vi "Teleop.vi"(0 "Call Context":T9) -> (6 "SubState 3":T4, 9 "SubState 4":T8, 11 "Loop 3 Data":T3, 14 "SubState 0":T4=enum."driver control", 15 "Loop 1 Data":T6, 16 "Loop 0 Data":T7, 17 "SubState 1":T4, 18 "Loop 2 Data":T5, 19 "SubState 2":T4)   [LabVIEW 2013]
uses:
  typedefs/subStates.ctl
  <vilib>/Rock Robotics/WPI/DriverStation/WPI_DriverStationDerivedRobotMode.ctl
  typedefs/singleUseSubstate.ctl
  typedefs/Loop Datatypes/Loop 0 Datatype.ctl
  typedefs/Loop Datatypes/Loop 1 Datatype.ctl
  typedefs/Loop Datatypes/Loop 2 Datatype.ctl
  typedefs/Loop Datatypes/Loop 3 Datatype.ctl
  <vilib>/Rock Robotics/WPI/Joystick/WPI_JoystickDevRef.ctl
  <vilib>/Rock Robotics/WPI/Joystick/WPI_JoystickDeviceEnum.ctl
  typedefs/fg_typedef.ctl
  typedefs/vision enable.ctl
  <vilib>/Rock Robotics/WPI/Joystick/WPI_JoystickGetSetRefNum.vi
panel:
  out "JS3":T1
  out "Drive to DC":bool
  out "JS1":T1
  out "JS2":T1
  out "Exit Value":i32=-1
  # "Loop Data and Substates"
  # "Drive Loop"
  # "State Machine Master Loop"
  # "Pickup/Passing Belts Loop"
  # "Pickup/Passing Arm Loop"
  # "Pneumatics Loop"
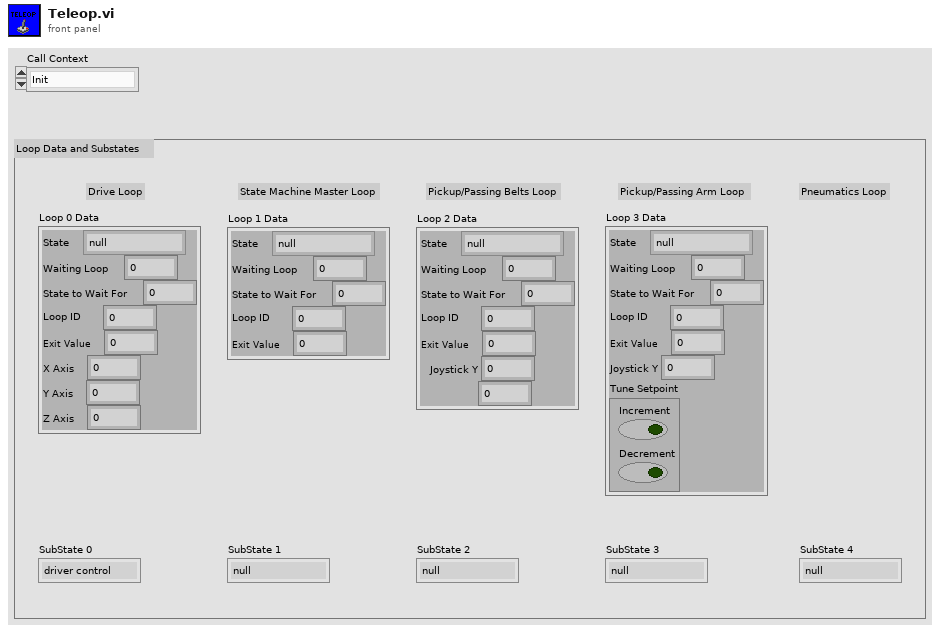
[diagram p1: front panel]
types:
  T1 = typedef "WPI_JoystickDevRef.ctl" = cluster{"Device":T2}
  T2 = typedef "WPI_JoystickDeviceEnum.ctl" = enum16{"USB 1", "USB 2", "USB 3", "USB 4", "Kinect 1", "Kinect 2"}
  T3 = typedef "Loop 3 Datatype.ctl" = cluster{"State":T4, "Waiting Loop":i32, "State to Wait For":i32, "Loop ID":i32, "Exit Value":i32, "Joystick Y":dbl, "Tune Setpoint":cluster{"Increment":bool, "Decrement":bool}}
  T4 = typedef "subStates.ctl" = enum16{"null", "wait", "driver control", "auto", "manual override", "hold position", "rotate", "pickup", "pass", "load", "goto shoot", "shoot high goal", "shoot low goal", "cancel arm", "cancel shooter", "end"}
  T5 = typedef "Loop 2 Datatype.ctl" = cluster{"State":T4, "Waiting Loop":i32, "State to Wait For":i32, "Loop ID":i32, "Exit Value":i32, "Joystick Y":dbl, "Joystick Z":dbl}
  T6 = typedef "Loop 1 Datatype.ctl" = cluster{"State":T4, "Waiting Loop":i32, "State to Wait For":i32, "Loop ID":i32, "Exit Value":i32}
  T7 = typedef "Loop 0 Datatype.ctl" = cluster{"State":T4, "Waiting Loop":i32, "State to Wait For":i32, "Loop ID":i32, "Exit Value":i32, "X Axis":dbl, "Y Axis":dbl, "Z Axis":dbl}
  T8 = typedef "singleUseSubstate.ctl" = enum16{"null", "wait", "shift high", "shift low", "extend shooter", "retract shooter", "latch", "unlatch"}
  T9 = typedef "WPI_DriverStationDerivedRobotMode.ctl" = enum16{"Init", "Execute", "Stop"}
  T10 = cluster{"axis 1 (x)":dbl, "axis 2 (y)":dbl, "axis 3 (throttle)":dbl, "axis 4":dbl, "axis 5":dbl, "axis 6":dbl}
  T11 = typedef "WPI_EncoderDevRef.ctl" = cluster{"DevStatus":errorcluster, "EncoderIndex":T12, "CounterIndex":T13, "DistancePerCount":dbl, "Decoding Type":T14}
  T12 = typedef "FPGA_EncoderIdx.ctl" = enum8{"Enc 0", "Enc 1", "Enc 2", "Enc 3", "Invalid"}
  T13 = typedef "FPGA_CounterCtrSystemIndex.ctl" = enum8{"Ctr 0", "Ctr 1", "Ctr 2", "Ctr 3", "Ctr 4", "Ctr 5", "Ctr 6", "Ctr 7", "Invalid"}
  T14 = typedef "WPI_EncoderType.ctl" = enum16{"1x", "2x", "4x"}
  T15 = typedef "vision enable.ctl" = enum16{"Enable", "Disable", "Stop"}
  T16 = typedef "fg_typedef.ctl" = enum16{"Get", "Set"}
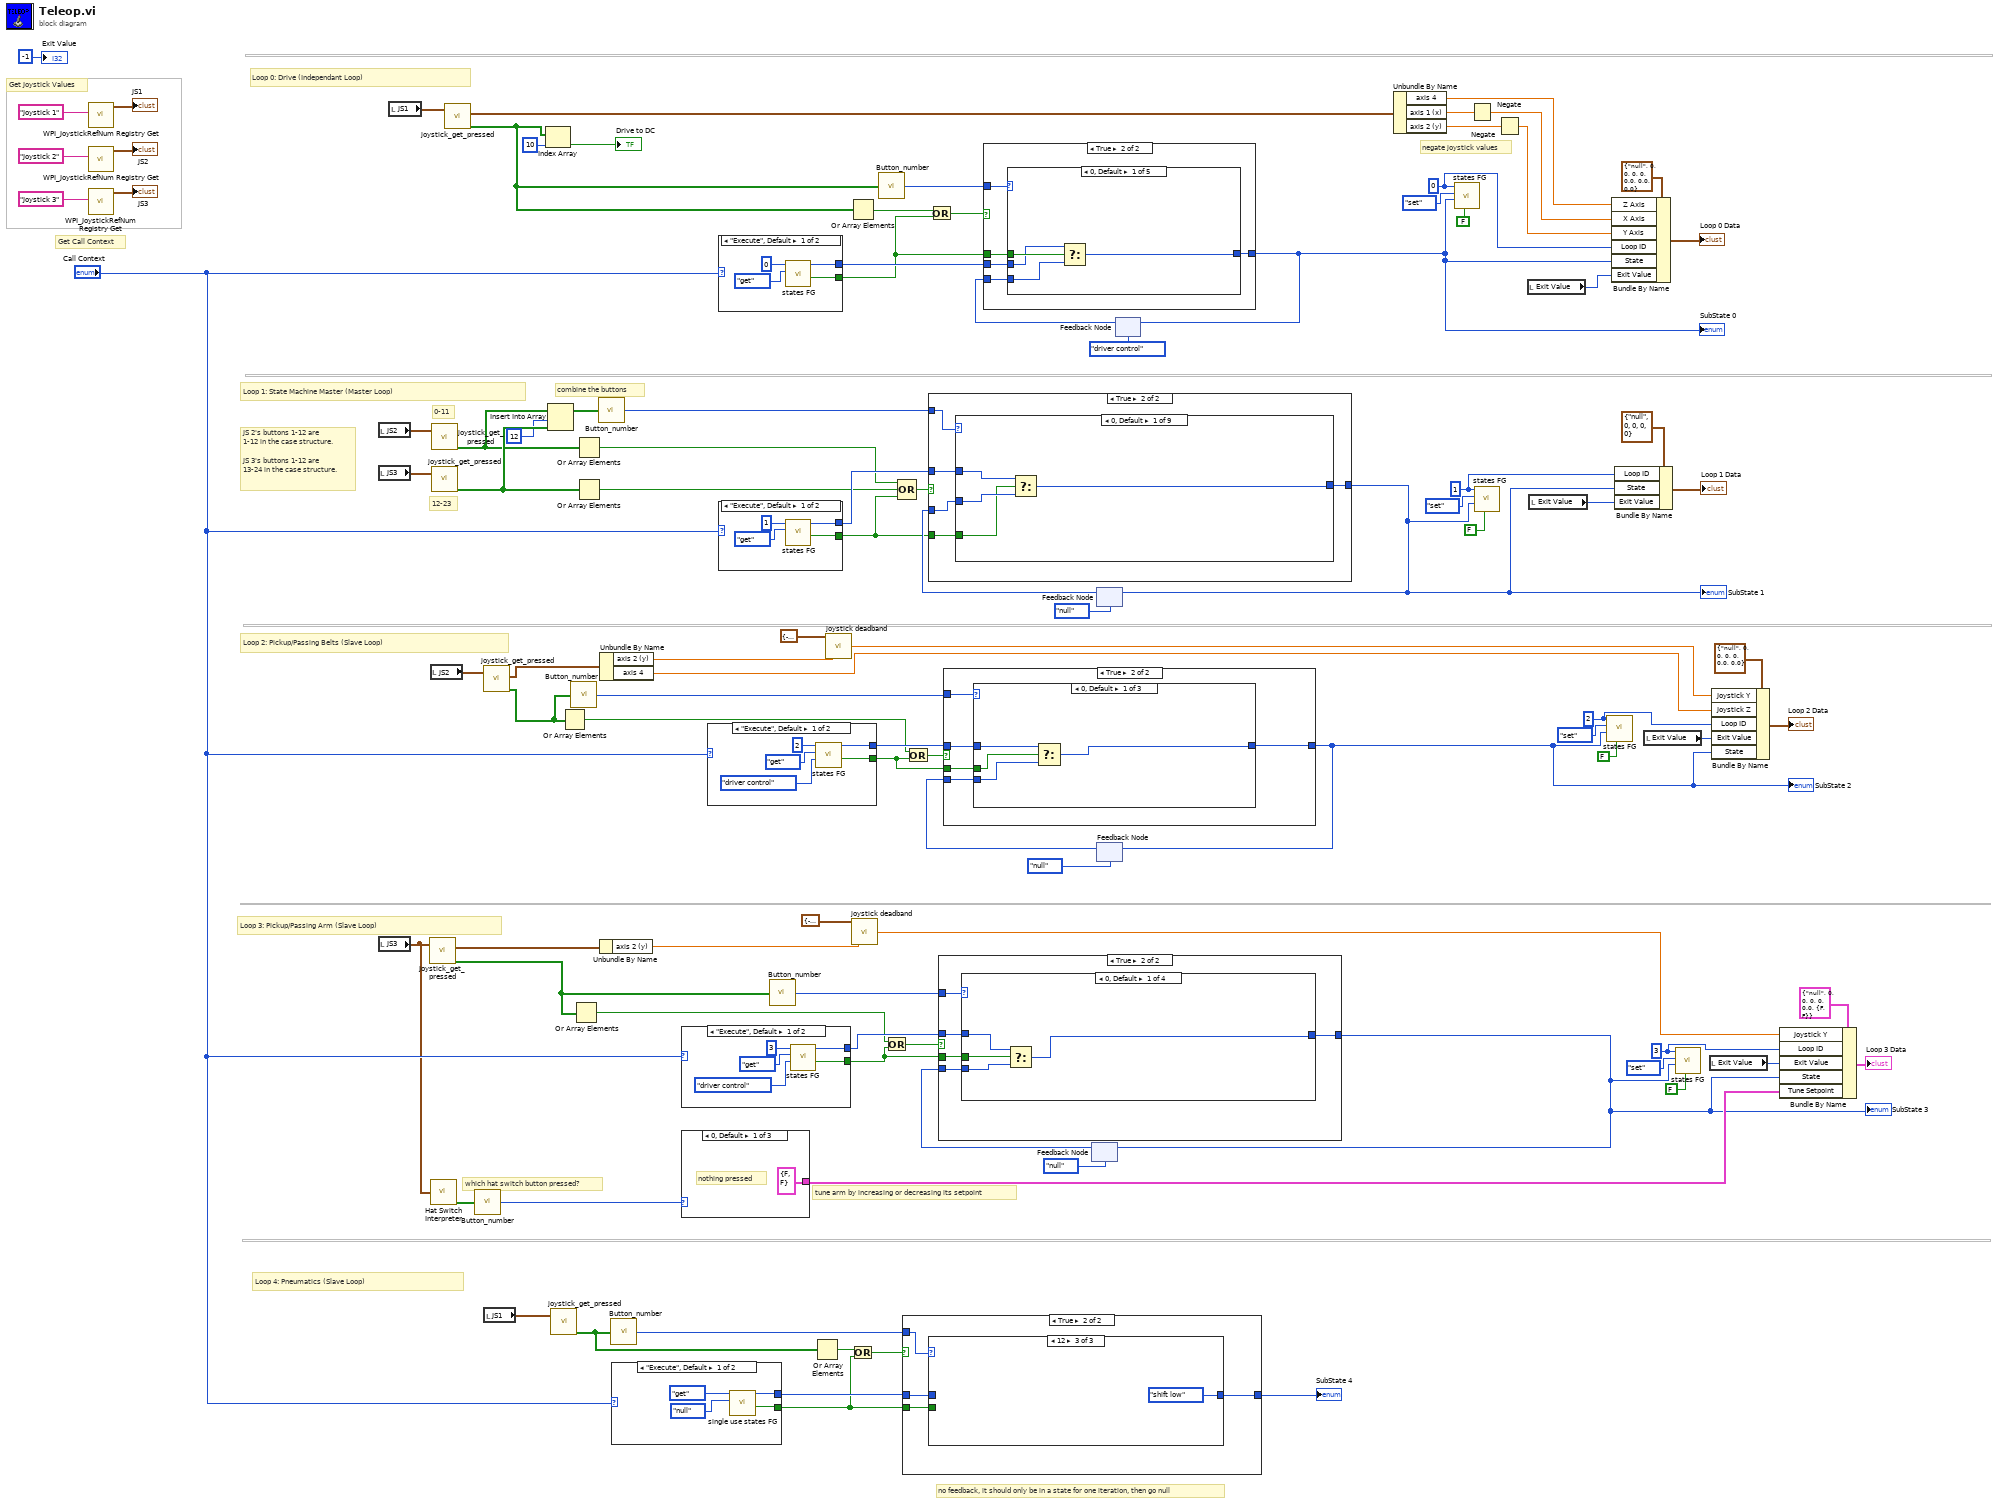
[diagram p0: block diagram]
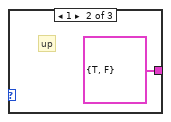
[diagram p2: hidden frame]
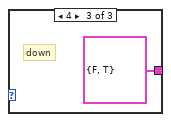
[diagram p3: hidden frame]
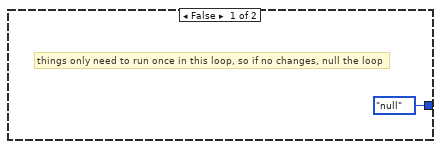
[diagram p4: hidden frame]
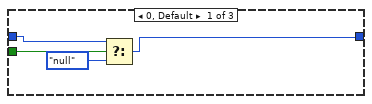
[diagram p5: hidden frame]
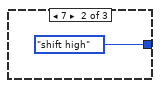
[diagram p6: hidden frame]
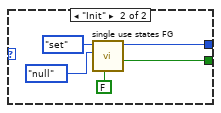
[diagram p7: hidden frame]
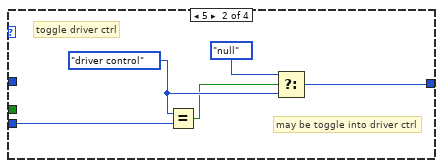
[diagram p9: hidden frame]
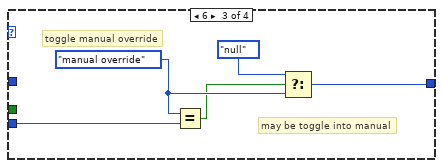
[diagram p10: hidden frame]
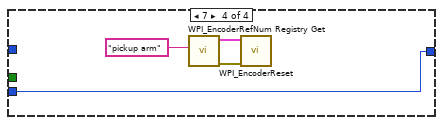
[diagram p11: hidden frame]
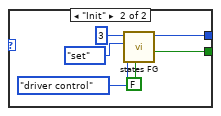
[diagram p12: hidden frame]
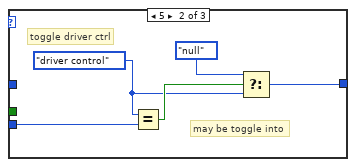
[diagram p14: hidden frame]
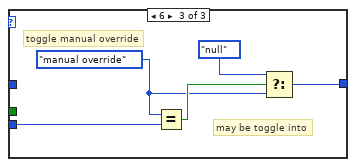
[diagram p15: hidden frame]
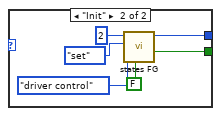
[diagram p16: hidden frame]
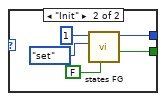
[diagram p17: hidden frame]
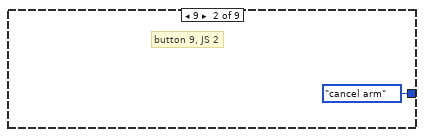
[diagram p19: hidden frame]
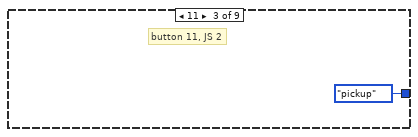
[diagram p20: hidden frame]
diagram:
  w77 = 3 ("Loop ID")
  w78 = 2 ("Loop ID")
  w87 = 1 ("Loop ID")
  w89 = 0 ("Loop ID")
  # "no feedback, it should only be in a state for one iteration, then go null"
  # "JS 2's buttons 1-12 are\n1-12 in the case structure.\n\nJS 3's buttons 1-12 are\n13-24 in the case structure."
  # "combine the buttons"
  # "12-23"
  # "0-11"
  # "tune arm by increasing or decreasing its setpoint"
  # "which hat switch button pressed?"
  # "negate joystick values"
  # "Get Call Context"
  # "Get Joystick Values"
  # "Loop 3: Pickup/Passing Arm (Slave Loop)"
  # "Loop 4: Pneumatics (Slave Loop)"
  # "Loop 2: Pickup/Passing Belts (Slave Loop)"
  # "Loop 1: State Machine Master (Master Loop)"
  # "Loop 0: Drive (Independant Loop)"
  n1 = call <vilib>:"WPI_JoystickRefNum Registry Get.vi"("refnum name"="Joystick 1") -> ("JoystickDevRef"=→"JS1":T1)  [unwired: 9 in, 1 out]
  n2 = call <vilib>:"WPI_JoystickRefNum Registry Get.vi"("refnum name"="Joystick 2") -> ("JoystickDevRef"=→"JS2":T1)  [unwired: 9 in, 1 out]
  n3 = call <vilib>:"WPI_JoystickRefNum Registry Get.vi"("refnum name"="Joystick 3") -> ("JoystickDevRef"=→"JS3":T1)  [unwired: 9 in, 1 out]
  n4 = local read "JS2"() -> (w56:T1)
  n5 = local read "JS3"() -> (w7:T1)
  n6 = local read "JS3"() -> (w20:T1)
  n7 = local read "JS1"() -> (w57:T1)
  n8 = call "joystick_get_pressed.vi"("JoystickDevRef 2"=w20) -> ("Axes"=w46:T10, "Buttons Pressed?"=w27:bool[])  [unwired: 1 in, 2 out]
  n9 = local read "JS2"() -> (w33:T1)
  n10 = call "Hat Switch Interpreter.vi"("JoystickDevRef"=w20) -> ("Buttons"=w19:bool[])  [unwired: 4 out]
  n11 = call "joystick_get_pressed.vi"("JoystickDevRef 2"=w56) -> ("Buttons Pressed?"=w3:bool[])  [unwired: 1 in, 3 out]
  n12 = call "joystick_get_pressed.vi"("JoystickDevRef 2"=w7) -> ("Buttons Pressed?"=w4:bool[])  [unwired: 1 in, 3 out]
  n13 = call "joystick_get_pressed.vi"("JoystickDevRef 2"=w57) -> ("Axes"=w61:T10, "Buttons Pressed?"=w39:bool[])  [unwired: 1 in, 2 out]
  n14 = call "Button_number.vi"("Button Array"=w19) -> ("Button Pressed"=w18:i32)
  n15 = call "joystick_get_pressed.vi"("JoystickDevRef 2"=w33) -> ("Axes"=w23:T10, "Buttons Pressed?"=w24:bool[])  [unwired: 1 in, 2 out]
  n16 = local read "JS1"() -> (w36:T1)
  n17 = Index Array(array=w39, index=10) -> (element=→"Drive to DC":bool)
  n18 = Insert Into Array(array=w3, index=12, new element=w4) -> (w1:bool[])
  n19 = call "joystick_get_pressed.vi"("JoystickDevRef 2"=w36) -> ("Buttons Pressed?"=w11:bool[])  [unwired: 1 in, 3 out]
  n20 = Or Array Elements(Boolean array=w24) -> (logical OR=w32:bool)
  n21 = call "Button_number.vi"("Button Array"=w24) -> ("Button Pressed"=w31:i32)
  n22 = Or Array Elements(Boolean array=w27) -> (logical OR=w45:bool)
  n23 = Or Array Elements(Boolean array=w3) -> (logical OR=w6:bool)
  n24 = Or Array Elements(Boolean array=w4) -> (logical OR=w5:bool)
  n25 = call "Button_number.vi"("Button Array"=w1) -> ("Button Pressed"=w50:i32)
  n26 = Unbundle By Name(w46) -> ("axis 2 (y)"=w42:dbl)
  n27 = Unbundle By Name(w23) -> ("axis 2 (y)"=w26:dbl, "axis 4"=w21:dbl)
  n28 = call "Button_number.vi"("Button Array"=w11) -> ("Button Pressed"=w10:i32)
  n29 = case shown="\"Execute\", Default" "Call Context" {
    tunnel: [w108 w111] -> w9
    tunnel: [w109 w110] -> w25
    frame "Execute", Default {
      n30 = call "single use states FG.vi"("substate"=singleUseSubstate."null" ("Enum"), "menu (get)"=enum16{"set", "get"}."get") -> ("exit out"=w108:bool, "substate out"=w109:T8)  [unwired: 6 in, 2 out]
    }
    frame "Init" {
      n31 = call "single use states FG.vi"("exit in"=FALSE, "substate"=singleUseSubstate."null", "menu (get)"=enum16{"set", "get"}."set") -> ("exit out"=w111:bool, "substate out"=w110:T8)  [unwired: 5 in, 2 out]
    }
  }
  n32 = case shown="\"Execute\", Default" "Call Context" {
    tunnel: [w117 w123] -> w43
    tunnel: [w115 w120] -> w75
    frame "Execute", Default {
      n33 = call "states FG.vi"("subState in"=subStates."driver control", "menu (get)"=enum16{"set", "get"}."get", "Loop ID"=3) -> ("exit out"=w117:bool, "subState out"=w115:T4)  [unwired: 5 in, 2 out]
    }
    frame "Init" {
      n34 = call "states FG.vi"("exit in"=FALSE, "subState in"=subStates."driver control", "menu (get)"=enum16{"set", "get"}."set", "Loop ID"=3) -> ("exit out"=w123:bool, "subState out"=w120:T4)  [unwired: 4 in, 2 out]
    }
  }
  n35 = case shown="0, Default" w18 {
    tunnel: [cluster{"Increment":bool, "Decrement":bool} {"Increment"=FALSE, "Decrement"=FALSE} cluster{"Increment":bool, "Decrement":bool} {"Increment"=TRUE, "Decrement"=FALSE} cluster{"Increment":bool, "Decrement":bool} {"Increment"=FALSE, "Decrement"=TRUE}] -> w16
    frame 0, Default {
      # "nothing pressed"
    }
    frame 1 {
      # "up"
    }
    frame 4 {
      # "down"
    }
  }
  n36 = case shown="\"Execute\", Default" "Call Context" {
    tunnel: [w131 w137] -> w48
    tunnel: [w129 w134] -> w94
    frame "Execute", Default {
      n37 = call "states FG.vi"("subState in"=subStates."driver control", "menu (get)"=enum16{"set", "get"}."get", "Loop ID"=2) -> ("exit out"=w131:bool, "subState out"=w129:T4)  [unwired: 5 in, 2 out]
    }
    frame "Init" {
      n38 = call "states FG.vi"("exit in"=FALSE, "subState in"=subStates."driver control", "menu (get)"=enum16{"set", "get"}."set", "Loop ID"=2) -> ("exit out"=w137:bool, "subState out"=w134:T4)  [unwired: 4 in, 2 out]
    }
  }
  n39 = case shown="\"Execute\", Default" "Call Context" {
    tunnel: [w141 w146] -> w54
    tunnel: [w140 w144] -> w92
    frame "Execute", Default {
      n40 = call "states FG.vi"("menu (get)"=enum16{"set", "get"}."get", "Loop ID"=0) -> ("exit out"=w141:bool, "subState out"=w140:T4)  [unwired: 6 in, 2 out]
    }
    frame "Init" {
      n41 = call "states FG.vi"("exit in"=FALSE, "menu (get)"=enum16{"set", "get"}."set", "Loop ID"=0) -> ("exit out"=w146:bool, "subState out"=w144:T4)  [unwired: 5 in, 2 out]
    }
  }
  n42 = case shown="\"Execute\", Default" "Call Context" {
    tunnel: [w150 w155] -> w51
    tunnel: [w149 w153] -> w91
    frame "Execute", Default {
      n43 = call "states FG.vi"("menu (get)"=enum16{"set", "get"}."get", "Loop ID"=1) -> ("exit out"=w150:bool, "subState out"=w149:T4)  [unwired: 6 in, 2 out]
    }
    frame "Init" {
      n44 = call "states FG.vi"("exit in"=FALSE, "menu (get)"=enum16{"set", "get"}."set", "Loop ID"=1) -> ("exit out"=w155:bool, "subState out"=w153:T4)  [unwired: 5 in, 2 out]
    }
  }
  n45 = call "Button_number.vi"("Button Array"=w27) -> ("Button Pressed"=w44:i32)
  n46 = Or Array Elements(Boolean array=w11) -> (logical OR=w12:bool)
  n47 = call "joystick deadband.vi"("Joystick In"=w26, "Deadband Range"=cluster{"Deadband Min":dbl, "Deadband Max":dbl} {"Deadband Min"=-0.05, "Deadband Max"=0.05}) -> ("Joystick Out"=w22:dbl)  [unwired: 4 in]
  n48 = Or Array Elements(Boolean array=w39) -> (logical OR=w55:bool)
  n49 = Or(x=w12, y=w9) -> (x .or. y?=w13:bool)
  n50 = call "joystick deadband.vi"("Joystick In"=w42, "Deadband Range"=cluster{"Deadband Min":dbl, "Deadband Max":dbl} {"Deadband Min"=-0.05, "Deadband Max"=0.05}) -> ("Joystick Out"=w17:dbl)  [unwired: 4 in]
  n51 = call "Button_number.vi"("Button Array"=w39) -> ("Button Pressed"=w60:i32)
  n52 = Or(x=w45, y=w43) -> (x .or. y?=w47:bool)
  n53 = Compound Arithmetic op=OR(w6, w5, w51) -> (w52:bool)
  n54 = case shown="True" w13 {
    tunnel: [singleUseSubstate."null" ("Enum") w159] -> w8
    tunnel: w25 -> [_ w160]
    tunnel: w10 -> [_ w161]
    tunnel: w9 -> [_ w162]
    frame False {
      # "things only need to run once in this loop, so if no changes, null the loop"
    }
    frame True {
      n55 = case shown="12" w161 {
        tunnel: w162 -> [w166 _ _]
        tunnel: w160 -> [w165 _ _]
        tunnel: [w164 singleUseSubstate."shift high" ("Enum") singleUseSubstate."shift low" ("Enum")] -> w159
        frame 0, Default {
          n56 = Select(t=w165, s=w166, f=singleUseSubstate."null") -> (s? t:f=w164:T8)
        }
        frame 7 {
        }
        frame 12 {
        }
      }
    }
  }
  "SubState 4" <- w8
  n57 = Or(x=w32, y=w48) -> (x .or. y?=w49:bool)
  n58 = Or(x=w55, y=w54) -> (x .or. y?=w53:bool)
  n59 = feedback #1(subStates."null" ("Drive SubState")) -> (w72:T4)
  n60 = case shown="True" w47 {
    tunnel: w72 -> [w169 w170]
    tunnel: [w169 w171] -> w15
    tunnel: w75 -> [_ w172]
    tunnel: w44 -> [_ w174]
    tunnel: w43 -> [_ w173]
    frame False {
      # "*yawn* nothing to do except wire through the previous state"
    }
    frame True {
      n61 = case shown="0, Default" w174 {
        tunnel: w173 -> [w178 _ _ _]
        tunnel: w170 -> [w177 w179 w184 w192]
        tunnel: w172 -> [w176 _ _ _]
        tunnel: [w175 w180 w185 w192] -> w171
        frame 0, Default {
          n62 = Select(t=w176, s=w178, f=w177) -> (s? t:f=w175:T4)
        }
        frame 5 {
          w182 = subStates."driver control" ("Drive SubState")
          # "may be toggle into driver ctrl"
          # "toggle driver ctrl"
          n63 = Equal?(x=w182, y=w179) -> (x = y?=w181:bool)
          n64 = Select(t=subStates."null", s=w181, f=w182) -> (s? t:f=w180:T4)
        }
        frame 6 {
          w188 = subStates."manual override" ("Drive SubState")
          # "may be toggle into manual"
          # "toggle manual override"
          n65 = Equal?(x=w188, y=w184) -> (x = y?=w186:bool)
          n66 = Select(t=subStates."null", s=w186, f=w188) -> (s? t:f=w185:T4)
        }
        frame 7 {
          n67 = call <vilib>:"WPI_EncoderRefNum Registry Get.vi"("refnum name"="pickup arm") -> ("error out"=w190:errorcluster, "EncoderDevRef"=w189:T11)  [unwired: 9 in]
          n68 = call <vilib>:"WPI_EncoderReset.vi"("error in (no error)"=w190, "EncoderDevRef"=w189) -> ()  [unwired: 8 in, 2 out]
        }
      }
    }
  }
  "SubState 3" <- w15
  n69 = feedback-in #1(w15) -> ()
  n70 = feedback #2(subStates."null" ("Drive SubState")) -> (w93:T4)
  n71 = case shown="True" w52 {
    tunnel: w93 -> [w193 w197]
    tunnel: [w193 w196] -> w62
    tunnel: w91 -> [_ w198]
    tunnel: w50 -> [_ w195]
    tunnel: w51 -> [_ w194]
    frame False {
      # "nothing pressed here, move along (wire through the previous state)"
    }
    frame True {
      n72 = case shown="0, Default" w195 {
        tunnel: w198 -> [w202 _ _ _ _ _ _ _ _]
        tunnel: w197 -> [w201 _ _ _ _ _ _ _ _]
        tunnel: [w200 subStates."cancel arm" ("Drive SubState") subStates."pickup" ("Drive SubState") subStates."pass" ("Drive SubState") subStates."shoot high goal" ("Drive SubState") subStates."load" ("Drive SubState") subStates."manual override" ("Drive SubState") subStates."shoot low goal" ("Drive SubState") subStates."cancel shooter" ("Drive SubState")] -> w196
        tunnel: w194 -> [w199 _ _ _ _ _ _ _ _]
        frame 0, Default {
          n73 = Select(t=w202, s=w199, f=w201) -> (s? t:f=w200:T4)
        }
        frame 9 {
          # "button 9, JS 2"
        }
        frame 11 {
          # "button 11, JS 2"
        }
        frame 12 {
          # "button 12, JS 2"
        }
        frame 13 {
          # "button 1, JS 3"
        }
        frame 14 {
          # "button 2, JS 3"
        }
        frame 20 {
          # "manual shoot"
          # "button 8, JS 3"
        }
        frame 23 {
          # "button 11, JS 3"
        }
        frame 24 {
          # "button 12, JS 3"
        }
      }
    }
  }
  "SubState 1" <- w62
  n74 = feedback-in #2(w62) -> ()
  n75 = feedback #3(subStates."null" ("Drive SubState")) -> (w97:T4)
  n76 = case shown="True" w49 {
    tunnel: w97 -> [w211 w213]
    tunnel: [w211 w212] -> w14
    tunnel: w94 -> [_ w214]
    tunnel: w31 -> [_ w216]
    tunnel: w48 -> [_ w215]
    frame False {
      # "nothing pressed, wire through last state"
    }
    frame True {
      n77 = case shown="0, Default" w216 {
        tunnel: w215 -> [w220 _ _]
        tunnel: w214 -> [w219 _ _]
        tunnel: w213 -> [w218 w225 w227]
        tunnel: [w217 w221 w226] -> w212
        frame 0, Default {
          n78 = Select(t=w219, s=w220, f=w218) -> (s? t:f=w217:T4)
        }
        frame 5 {
          w223 = subStates."driver control" ("Drive SubState")
          # "may be toggle into"
          # "toggle driver ctrl"
          n79 = Equal?(x=w223, y=w225) -> (x = y?=w224:bool)
          n80 = Select(t=subStates."null", s=w224, f=w223) -> (s? t:f=w221:T4)
        }
        frame 6 {
          w228 = subStates."manual override" ("Drive SubState")
          # "may be toggle into"
          # "toggle manual override"
          n81 = Equal?(x=w228, y=w227) -> (x = y?=w230:bool)
          n82 = Select(t=subStates."null", s=w230, f=w228) -> (s? t:f=w226:T4)
        }
      }
    }
  }
  "SubState 2" <- w14
  n83 = feedback-in #3(w14) -> ()
  n84 = feedback #4(subStates."driver control" ("Drive SubState")) -> (w99:T4)
  n85 = case shown="True" w53 {
    tunnel: w99 -> [w231 w233]
    tunnel: [w231 w232] -> w35
    tunnel: w92 -> [_ w234]
    tunnel: w60 -> [_ w236]
    tunnel: w54 -> [_ w235]
    frame False {
      # "keep current state, no change necessary"
    }
    frame True {
      n86 = case shown="0, Default" w236 {
        tunnel: w235 -> [w240 _ _ _ _]
        tunnel: w234 -> [w239 _ _ _ _]
        tunnel: w233 -> [w238 w245 w253 _ _]
        tunnel: [w237 w241 w253 subStates."goto shoot" ("Drive SubState") subStates."driver control" ("Drive SubState")] -> w232
        frame 0, Default {
          n87 = Select(t=w239, s=w240, f=w238) -> (s? t:f=w237:T4)
        }
        frame 1 {
          w242 = subStates."hold position" ("x")
          # "button 1, hold position toggle"
          n88 = Equal?(x=w242, y=w245) -> (x = y?=w244:bool)
          n89 = Select(t=subStates."driver control" ("Drive SubState"), s=w244, f=w242) -> (s? t:f=w241:T4)
        }
        frame 8 {
          w248 = vision_enable."Enable" ("y")
          # "toggle vision"
          n90 = call "vision_fg.vi"("Menu"=fg_typedef."Get") -> ("State Out"=w250:T15)  [unwired: 2 in, 1 out]
          n91 = Equal?(x=w250, y=w248) -> (x = y?=w249:bool)
          n92 = Select(t=vision_enable."Disable" ("y"), s=w249, f=w248) -> (s? t:f=w246:T15)
          n93 = call "vision_fg.vi"("Action"=w246, "Menu"=fg_typedef."Set") -> ()  [unwired: 1 in, 2 out]
        }
        frame 10 {
          # "go to shoot location"
          n94 = call "vision_fg.vi"("Action"=vision_enable."Enable", "Menu"=fg_typedef."Set") -> ()  [unwired: 1 in, 2 out]
        }
        frame 11 {
          # "put robot drive in driver control"
          n95 = call "vision_fg.vi"("Action"=vision_enable."Disable", "Menu"=fg_typedef."Set") -> ()  [unwired: 1 in, 2 out]
        }
      }
    }
  }
  "SubState 0" <- w35
  n96 = feedback-in #4(w35) -> ()
  n97 = Unbundle By Name(w61) -> ("axis 4"=w40:dbl, "axis 1 (x)"=w66:dbl, "axis 2 (y)"=w65:dbl)
  n98 = call "states FG.vi"("exit in"=FALSE, "subState in"=w35, "menu (get)"=enum16{"set", "get"}."set", "Loop ID"=w89) -> ()  [unwired: 4 in, 4 out]
  n99 = Negate(x=w66) -> (-x=w64:dbl)
  n100 = call "states FG.vi"("exit in"=FALSE, "subState in"=w62, "menu (get)"=enum16{"set", "get"}."set", "Loop ID"=w87) -> ()  [unwired: 4 in, 4 out]
  n101 = Negate(x=w65) -> (-x=w63:dbl)
  n102 = local read "Exit Value"() -> (w85:i32)
  n103 = local read "Exit Value"() -> (w84:i32)
  n104 = call "states FG.vi"("exit in"=FALSE, "subState in"=w14, "menu (get)"=enum16{"set", "get"}."set", "Loop ID"=w78) -> ()  [unwired: 4 in, 4 out]
  n105 = Bundle By Name(cluster=T7 {"State"=enum."null", "Waiting Loop"=0, "State to Wait For"=0, "Loop ID"=0, "Exit Value"=0, "X Axis"=0.0, "Y Axis"=0.0, "Z Axis"=0.0} ("Cluster"), "Z Axis"=w40, "X Axis"=w64, "Y Axis"=w63, "Loop ID"=w89, "State"=w35, "Exit Value"=w85) -> (→"Loop 0 Data":T7)
  n106 = Bundle By Name(cluster=T6 {"State"=enum."null", "Waiting Loop"=0, "State to Wait For"=0, "Loop ID"=0, "Exit Value"=0} ("Cluster"), "Loop ID"=w87, "State"=w62, "Exit Value"=w84) -> (→"Loop 1 Data":T6)
  n107 = local read "Exit Value"() -> (w79:i32)
  n108 = call "states FG.vi"("exit in"=FALSE, "subState in"=w15, "menu (get)"=enum16{"set", "get"}."set", "Loop ID"=w77) -> ()  [unwired: 4 in, 4 out]
  n109 = local read "Exit Value"() -> (w76:i32)
  n110 = Bundle By Name(cluster=T5 {"State"=enum."null", "Waiting Loop"=0, "State to Wait For"=0, "Loop ID"=0, "Exit Value"=0, "Joystick Y"=0.0, "Joystick Z"=0.0} ("Loop 2 Data"), "Joystick Y"=w22, "Joystick Z"=w21, "Loop ID"=w78, "Exit Value"=w79, "State"=w14) -> (→"Loop 2 Data":T5)
  n111 = Bundle By Name(cluster=T3 {"State"=enum."null", "Waiting Loop"=0, "State to Wait For"=0, "Loop ID"=0, "Exit Value"=0, "Joystick Y"=0.0, "Tune Setpoint"={"Increment"=FALSE, "Decrement"=FALSE}} ("Loop 3 Data"), "Joystick Y"=w17, "Loop ID"=w77, "Exit Value"=w76, "State"=w15, "Tune Setpoint"=w16) -> (→"Loop 3 Data":T3)
  "Exit Value" <- -1 ("Exit Value")
